vi "string to lat_lon.vi"(7 "magnetic variation?":bool, 9 "direction string":string, 10 "numeric string for lat/lon":string) -> (2 "composite value":dbl)   [LabVIEW 2011, in "u-blox 5 Series.lvlib"]
uses:
  u-blox 5 Series.lvlib
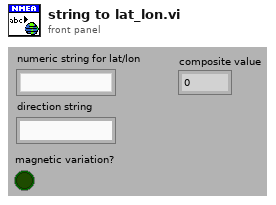
[diagram p1: front panel]
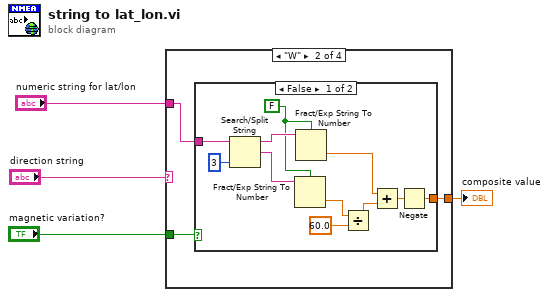
[diagram p0: block diagram]
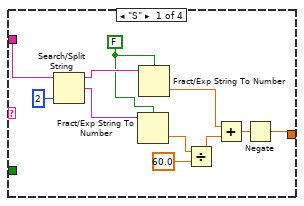
[diagram p2: hidden frame]
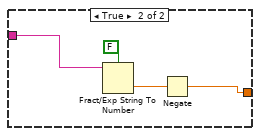
[diagram p3: hidden frame]
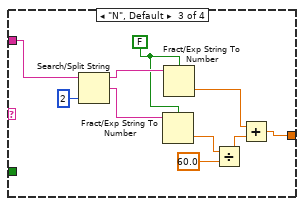
[diagram p4: hidden frame]
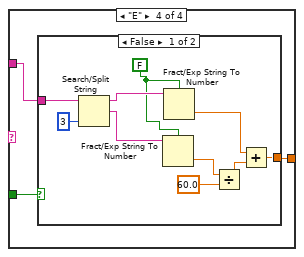
[diagram p5: hidden frame]
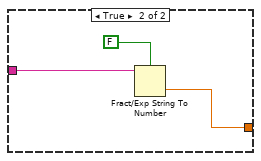
[diagram p6: hidden frame]
diagram:
  n1 = case shown="\"W\"" "direction string" {
    tunnel: "numeric string for lat/lon" -> [w8 w18 w43 w46]
    tunnel: [w6 w17 w35 w45] -> w2
    tunnel: "magnetic variation?" -> [_ w16 _ w44]
    frame "S" {
      w5 = FALSE ("use system decimal point (T)")
      n2 = Search/Split String(string=w8, offset (0)=2) -> (substring before match=w14:string, match + rest of string=w13:string)  [unwired: 2 out]
      n3 = Fract/Exp String To Number(use system decimal point (T)=w5, string=w13) -> (number=w12:dbl)  [unwired: 3 out]
      n4 = Fract/Exp String To Number(use system decimal point (T)=w5, string=w14) -> (number=w9:dbl)  [unwired: 3 out]
      n5 = Divide(x=w12, y=60.0) -> (x/y=w10:dbl)
      n6 = Add(x=w9, y=w10) -> (x+y=w7:dbl)
      n7 = Negate(x=w7) -> (-x=w6:dbl)
    }
    frame "W" {
      n8 = case shown="False" w16 {
        tunnel: w18 -> [w22 w33]
        tunnel: [w20 w31] -> w17
        frame False {
          w19 = FALSE ("use system decimal point (T)")
          n9 = Search/Split String(string=w22, offset (0)=3) -> (substring before match=w28:string, match + rest of string=w27:string)  [unwired: 2 out]
          n10 = Fract/Exp String To Number(use system decimal point (T)=w19, string=w27) -> (number=w26:dbl)  [unwired: 3 out]
          n11 = Fract/Exp String To Number(use system decimal point (T)=w19, string=w28) -> (number=w23:dbl)  [unwired: 3 out]
          n12 = Divide(x=w26, y=60.0) -> (x/y=w24:dbl)
          n13 = Add(x=w23, y=w24) -> (x+y=w21:dbl)
          n14 = Negate(x=w21) -> (-x=w20:dbl)
        }
        frame True {
          n15 = Fract/Exp String To Number(use system decimal point (T)=FALSE, string=w33) -> (number=w32:dbl)  [unwired: 3 out]
          n16 = Negate(x=w32) -> (-x=w31:dbl)
        }
      }
    }
    frame "N", Default {
      w34 = FALSE ("use system decimal point (T)")
      n17 = Search/Split String(string=w43, offset (0)=2) -> (substring before match=w41:string, match + rest of string=w40:string)  [unwired: 2 out]
      n18 = Fract/Exp String To Number(use system decimal point (T)=w34, string=w40) -> (number=w39:dbl)  [unwired: 3 out]
      n19 = Fract/Exp String To Number(use system decimal point (T)=w34, string=w41) -> (number=w36:dbl)  [unwired: 3 out]
      n20 = Divide(x=w39, y=60.0) -> (x/y=w37:dbl)
      n21 = Add(x=w36, y=w37) -> (x+y=w35:dbl)
    }
    frame "E" {
      n22 = case shown="False" w44 {
        tunnel: w46 -> [w56 w59]
        tunnel: [w48 w58] -> w45
        frame False {
          w47 = FALSE ("use system decimal point (T)")
          n23 = Search/Split String(string=w56, offset (0)=3) -> (substring before match=w54:string, match + rest of string=w53:string)  [unwired: 2 out]
          n24 = Fract/Exp String To Number(use system decimal point (T)=w47, string=w53) -> (number=w52:dbl)  [unwired: 3 out]
          n25 = Fract/Exp String To Number(use system decimal point (T)=w47, string=w54) -> (number=w49:dbl)  [unwired: 3 out]
          n26 = Divide(x=w52, y=60.0) -> (x/y=w50:dbl)
          n27 = Add(x=w49, y=w50) -> (x+y=w48:dbl)
        }
        frame True {
          n28 = Fract/Exp String To Number(use system decimal point (T)=FALSE, string=w59) -> (number=w58:dbl)  [unwired: 3 out]
        }
      }
    }
  }
  "composite value" <- w2
